vi "Init.vi"(8 "error in (no error)":errorcluster, 11 "Key Sequence":T1) -> (0 "error out":errorcluster, 3 "TriggerHotkeyByKeySequence out":refnum<class "TriggerHotkeyByKeySequence.lvclass">)   [LabVIEW 2020, in "obs-websocket.lvlib" / "TriggerHotkeyByKeySequence.lvclass"]
uses:
  TriggerHotkeyByKeySequence.lvclass
  TriggerHotkeyByKeySequence.lvclass/TriggerHotkeyByKeySequence.ctl
  OBS Key.ctl
  obs-websocket.lvlib
  Key Sequence.ctl
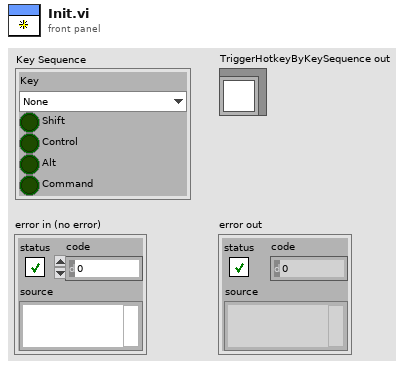
[diagram p1: front panel]
types:
  T1 = typedef "obs-websocket.lvlib/Key Sequence.ctl" = cluster{"Key":T2, "Shift":bool, "Control":bool, "Alt":bool, "Command":bool}
  T2 = typedef "obs-websocket.lvlib/OBS Key.ctl" = enum16{"None", "Return", "Enter", "Escape", "Tab", "Backtab", "Backspace", "Insert", "Delete", "Pause", "Print", "SysReq", "Clear", "Home", "End", "Left", "Up", "Right", "Down", "PageUp", "PageDown", "Shift", "Control", "Meta", "Alt", "AltGr", "Capslock", "Numlock", "Scrolllock", "F1", "F2", "F3", "F4", "F5", "F6", "F7", "F8", "F9", "F10", "F11", "F12", "F13", "F14", "F15", "F16", "F17", "F18", "F19", "F20", "F21", "F22", "F23", "F24", "F25", "F26", "F27", "F28", "F29", "F30", "F31", "F32", "F33", "F34", "F35", "Menu", "Hyper_L", "Hyper_R", "Help", "Direction_L", "Direction_R", "Space", "Exclam", "QuoteDbl", "NumberSign", "Dollar", "Percent", "Ampersand", "Apostrophe", "ParenLeft", "ParenRight", "Asterisk", "Plus", "Comma", "Minus", "Period", "Slash", "0", "1", "2", "3", "4", "5", "6", "7", "8", "9", "NumEqual", "NumAsterisk", "NumPlus", "NumComma", "NumMinus", "NumPeriod", "NumSlash", "Num0", "Num1", "Num2", "Num3", "Num4", "Num5", "Num6", "Num7", "Num8", "Num9", "Colon", "Semicolon", "Quote", "Less", "Equal", "Greater", "Question", "At", "A", "B", "C", "D", "E", "F", "G", "H", "I", "J", "K", "L", "M", "N", "O", "P", "Q", "R", "S", "T", "U", "V", "W", "X", "Y", "Z", "BracketLeft", "Backslash", "BracketRight", "AsciiCircum", "Underscore", "QuoteLeft", "BraceLeft", "Bar", "BraceRight", "AsciiTilde", "NoBreakSpace", "ExclamDown", "Cent", "Sterling", "Currency", "Yen", "Brokenbar", "Section", "Diaresis", "Copyright", "OrdFeminine", "GuillemotLeft", "NotSign", "Hyphen", "Registered", "Macron", "Degree", "PlusMinus", "TwoSuperior", "ThreeSuperior", "Acute", "Mu", "Paragraph", "PeriodCentered", "Cedilla", "OneSuperior", "Masculine", "GuillemotRight", "OneQuarter", "OneHalf", "ThreeQuarters", "QuestionDown", "Agrave", "AAcute", "ACircumflex", "ATilde", "ADiaresis", "ARing", "AE", "CCedilla", "EGrave", "EAcute", "ECircumflex", "EDiaresis", "IGrave", "IAcute", "ICircumflex", "IDiaresis", "Eth", "NTilde", "OGrave", "OAcute", "OCircumflex", "OTilde", "ODiaresis", "Multiply", "OOblique", "UGrave", "UAcute", "UCircumflex", "UDiaresis", "YAcute", "Thorn", "SSharp", "Division", "YDiaresis", "Multi_Key", "CodeInput", "SingleCandidate", "MultipleCandidate", "PreviousCandidate", "Mode_Switch", "Kanji", "Muhenkan", "Henkan", "Romaji", "Hiragana", "Katakana", "Hiragana_Katakana", "Zenkaku", "Hankaku", "Zenkaku_Hankaku", "Touroku", "Massyo", "Kana_Lock", "Kana_Shift", "Eisu_Shift", "Eisu_Toggle", "Hangul", "Hangul_Start", "Hangul_End", "Hangul_Hanja", "Hangul_Jamo", "Hangul_Romaja", "Hangul_Jeonja", "Hangul_Banja", "Hangul_Prehanja", "Hangul_Posthanja", "Hangul_Special", "Dead_Grave", "Dead_Acute", "Dead_Circumflex", "Dead_Tilde", "Dead_Macron", "Dead_Breve", "Dead_AboveDot", "Dead_Diaresis", "Dead_AboveRing", "Dead_DoubleAcute", "Dead_Caron", "Dead_Cedilla", "Dead_Ogonek", "Dead_Iota", "Dead_Voiced_Sound", "Dead_Semivoiced_Sound", "Dead_BelowDot", "Dead_Hook", "Dead_Horn", "Back", "Forward", "Stop", "Refresh", "VolumeDown", "VolumeMute", "VolumeUp", "BassBoost", "BassUp", "BassDown", "TrebleUp", "TrebleDown", "MediaPlay", "MediaStop", "MediaPrevious", "MediaNext", "MediaRecord", "MediaPause", "MediaTogglePlayPause", "Homepage", "Favorites", "Search", "Standby", "OpenURL", "LaunchMail", "LaunchMedia", "Launch0", "Launch1", "Launch2", "Launch3", "Launch4", "Launch5", "Launch6", "Launch7", "Launch8", "Launch9", "LaunchA", "LaunchB", "LaunchC", "LaunchD", "LaunchE", "LaunchF", "LaunchG", "LaunchH", "MonBrightnessUp", "MonBrightnessDown", "KeyboardLightOnOff", "KeyboardBrightnessUp", "KeyboardBrightnessDown", "Poweroff", "Wakeup", "Eject", "Screensaver", "WWW", "Memo", "Lightbulb", "Shop", "History", "AddFavorite", "Hotlinks", "BrightnessAdjust", "Finance", "Community", "AudioRewind", "BackForward", "ApplicationLeft", "ApplicationRight", "Book", "CD", "Calculator", "TodoList", "ClearGrab", "Close", "Copy", "Cut", "Display", "DOS", "Documents", "Excel", "Explorer", "Game", "Go", "ITouch", "Logoff", "Market", "Meeting", "MenuKB", "MenuPB", "MySites", "News", "OfficeHome", "Option", "Paste", "Phone", "Calendar", "Reply", "Reload", "RotateWindows", "RotationPB", "RotationKB", "Save", "Send", "Spell", "SplitScreen", "Support", "TakePane", "Terminal", "Tools", "Travel", "Video", "Word", "Xfer", "ZoomIn", "ZoomOut", "Away", "Messenger", "Webcam", "MailForward", "Pictures", "Music", "Battery", "Bluetooth", "WLan", "UWB", "AudioForward", "AudioRepeat", "AudioRandomPlay", "Subtitle", "AudioCycleTrack", "Time", "Hibernate", "View", "TopMenu", "Powerdown", "Suspend", "ContrastAdjust", "MediaLast", "Call", "Camera", "CameraFocus", "Context1", "Context2", "Context3", "Context4", "Flip", "Hangup", "No", "Select", "Yes", "ToggleCallHangup", "VoiceDial", "LastNumberRedial", "Execute", "Printer", "Play", "Sleep", "Zoom", "Cancel", "Mouse1", "Mouse2", "Mouse3", "Mouse4", "Mouse5", "Mouse6", "Mouse7", "Mouse8", "Mouse9", "Mouse10", "Mouse11", "Mouse12", "Mouse13", "Mouse14", "Mouse15", "Mouse16", "Mouse17", "Mouse18", "Mouse19", "Mouse20", "Mouse21", "Mouse22", "Mouse23", "Mouse24", "Mouse25", "Mouse26", "Mouse27", "Mouse28", "Mouse29", "Backslash_RT102", "Open", "Find", "Redo", "Undo", "Front", "Props"}
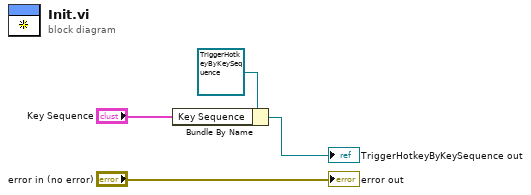
[diagram p0: block diagram]
diagram:
  n1 = Bundle By Name(cluster=refnum<class "TriggerHotkeyByKeySequence.lvclass"> refnum ("TriggerHotkeyByKeySequence in"), "Key Sequence"="Key Sequence") -> (→"TriggerHotkeyByKeySequence out":refnum<class "TriggerHotkeyByKeySequence.lvclass">)
  "error out" <- "error in (no error)"
